vi "Configure Averaging.vi"(7 "Enable Averaging (T: Enable)":bool=TRUE, 8 "error in (no error)":errorcluster, 9 "Averaging Count (8: Count 8)":i32(ring)=8 items=["Count 8"=8, "Count 16"=16, "Count 32"=32, "Count 64"=64], 10 "Averaging Type (0: Exponent)":i32(ring) items=["Exponent", "Linear"], 11 "VISA resource name":refnum<visa-resource-name>) -> (0 "error out":errorcluster, 3 "VISA resource name out":refnum<visa-resource-name>)   [LabVIEW 2019, in "Yokogawa WT300 Series.lvlib"]
doc: "Configures the averaging features."
uses:
  Yokogawa WT300 Series.lvlib
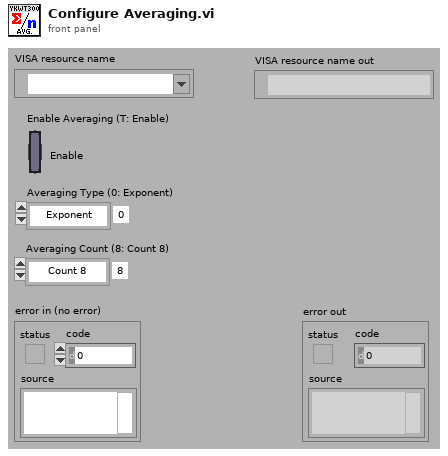
[diagram p1: front panel]
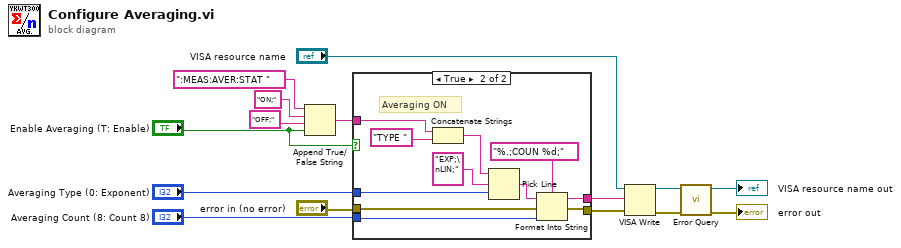
[diagram p0: block diagram]
diagram:
  n1 = Append True/False String ("True/False 文字列を追加")(1:"Enable Averaging (T: Enable)", 2:"OFF;", 3:"ON;", 4:":MEAS:AVER:STAT " ("¶ñi\"\"j")) -> (0:w3:string)
  n2 = case "ケースストラクチャ" shown="True" "Enable Averaging (T: Enable)" {
    tunnel: "Averaging Count (8: Count 8)" -> [_ w27]
    tunnel: "error in (no error)" -> [w17 w26]
    tunnel: [w16 w25] -> w9
    tunnel: [w17 w18] -> w8
    tunnel: w3 -> [w16 w23]
    tunnel: "Averaging Type (0: Exponent)" -> [_ w20]
    frame False {
      # "Averaging OFF"
    }
    frame True {
      # "Averaging ON"
      n3 = Concatenate Strings(w23, "TYPE ") -> (w21:string)
      n4 = Pick Line ("ライン選択")(string ("")=w21, multi-line string="EXP;\nLIN;" ("複数行文字列"), line index=w20) -> (output string=w19:string)
      n5 = Format Into String ("文字列にフォーマット")(format string="%.;COUN %d;" ("形式文字列"), initial string=w19, error in=w26, w27) -> (resulting string=w25:string, error out=w18:errorcluster)
    }
  }
  n6 = VISA Write ("VISA書き込み")(VISA resource name="VISA resource name", write buffer=w9, error in (no error)=w8) -> (VISA resource name out=w15:refnum<visa-resource-name>, error out=w14:errorcluster)  [unwired: 1 out]
  n7 = call "Error Query.vi"("error in (no error)"=w14, "VISA resource name"=w15) -> ("error out"=→"error out":errorcluster, "VISA resource name out"=→"VISA resource name out":refnum<visa-resource-name>)  [unwired: 6 in, 2 out]
